vi "IO Monitor Tester.vi"() -> ()   [LabVIEW 2022 SP3]
uses:
  Class 3/DAQ View.lvclass
  abstract IO Factory/abstract IO Factory.lvclass
  3e9cc303-48d4-40e1-83e6-25e531503efb.vi
  DAQ Controller/DAQ Controller.lvclass
  C:/XY Stage/IO Monitor/DAQ API/DAQ API.lvclass
  <vilib>/Utility/LVClass/Get LV Class Default Value.vi
  XY Stage/Framework/Read Configs/Read Configs Sections.lvlib
panel:
  in  "stop":bool
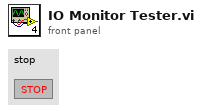
[diagram p1: front panel]
types:
  T1 = typedef "Read Configs Sections.lvlib/Section Data.ctl" = cluster{"Path":path, "Section":string}
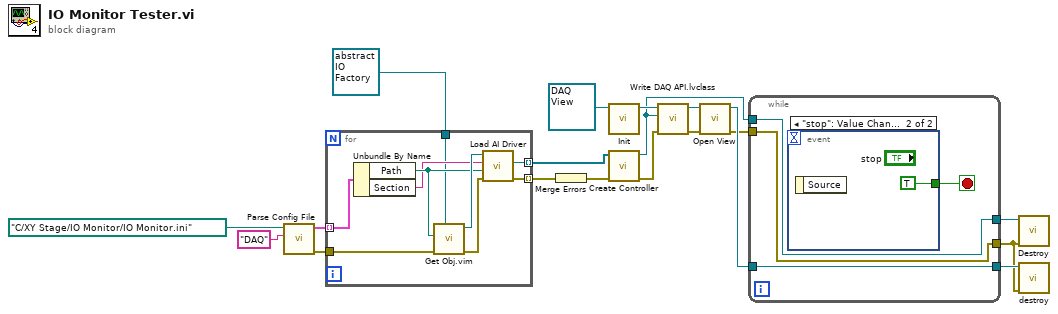
[diagram p0: block diagram]
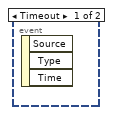
[diagram p2: hidden frame]
diagram:
  n1 = call "Parse Config File.vi"("Section"="DAQ", "Config Path"=path "C:/XY Stage/IO Monitor/IO Monitor.ini") -> ("error out"=w16:errorcluster, "Array"=w19:T1[])  [unwired: 8 in]
  n2 = for {
    tunnel: w19 -> [w28] mode=indexing
    tunnel: w16 -> [w27]
    tunnel: [w23] -> w15 mode=indexing
    tunnel: [w21] -> w7 mode=indexing
    tunnel: refnum<class "abstract IO Factory.lvclass"> refnum ("abstract IO Factory.lvclass") -> [w20]
    n3 = Unbundle By Name(w28) -> ("Path"=w25:path, "Section"=w24:string)
    n4 = call "Get Obj.vim"("LabVIEW Object 2"=w20, "error in (no error)"=w27, "Path"=w25) -> ("error out"=w22:errorcluster, "LabVIEW Object"=w26:refnum<class "abstract IO Factory.lvclass">)  [unwired: 7 in]
    n5 = call-dynamic "Load AI Driver.vi"("error in (no error)"=w22, "Config Path"=w25, "Section"=w24, "abstract IO Factory in"=w26) -> ("error out"=w21:errorcluster, "AI Driver.lvclass"=w23:refnum<class "AI Driver.lvclass">)  [unwired: 6 in]
  }
  n6 = Merge Errors(w7) -> (w6:errorcluster)
  n7 = call-dynamic "Init.vi"("DAQ View in"=refnum<class "DAQ View.lvclass"> refnum) -> ("DAQ View out"=w12:refnum<class "DAQ View.lvclass">)  [unwired: 9 in, 1 out]
  n8 = call "Create Controller.vi"("error in (no error)"=w6, "AI Driver"=w15) -> ("error out"=w5:errorcluster, "DAQ Controller out"=w11:refnum<class "DAQ Controller.lvclass">)  [unwired: 8 in]
  n9 = call "Write DAQ API.lvclass.vi"("error in (no error)"=w5, "DAQ API.lvclass"=w11, "In"=w12) -> ("error out"=w4:errorcluster, "Out"=w10:refnum<class "DAQ View.lvclass">)  [unwired: 7 in]
  n10 = call-dynamic "Open View.vi"("error in (no error)"=w4, "base view in"=w10) -> ("error out"=w3:errorcluster, "base view out"=w9:refnum<class "DAQ View.lvclass">)  [unwired: 8 in]
  n11 = while {
    tunnel: w11 -> [w31]
    tunnel: [w31] -> w14
    tunnel: w9 -> [w30]
    tunnel: [w30] -> w8
    tunnel: w3 -> [w29]
    tunnel: [w29] -> w2
    stop <- w32 stop-if-true
    n12 = event shown="[1] \"stop\": Value Change" {
      selector: _ -> [_ _]
      dyn-events: _ -> [_ _]
      timeout: _ -> [_ _]
      tunnel: [_ TRUE] -> w32
      event Timeout {
        n13 = event-data() -> ()  [unwired: 1 in, 3 out]
      }
      event "stop": Value Change {
        n14 = event-data() -> ()  [unwired: 1 in, 1 out]
      }
    }
  }
  n15 = call "Destroy.vi"("error in (no error)"=w2, "DAQ Controller in"=w14) -> ()  [unwired: 8 in, 2 out]
  n16 = call-dynamic "destroy.vi"("error in (no error)"=w2, "DAQ View in"=w8) -> ()  [unwired: 8 in, 2 out]
